vi "save_tiff.vi"(9 "image_info":T1={"file_path"=path "", "file_name"="", "image"=[], "image_size_xy"={"image_size_x_um"=1.0, "image_size_y_um"=1.0}, "pixel_dwell_time_ms"=1.0, "Laser_power_mW"=1.0, "pixel_size"=0.0, "tile_ij"={"tile_i"=0, "tile_j"=0}, "Objective"="", "ColorMarkers"=[], "timestamp"=timestamp(0 s since 1904-01-01), "micro-position-xyz"={"micro-position_x_mm"=1.0, "micro-position_y_mm"=1.0, "micro-position_z_mm"=1.0}, "zero_xyz"={"zero_x_mm"=0.0, "zero_y_mm"=0.0, "zero_z_mm"=0.0}, "nano-position-xyz"={"nano-position_x_V"=1.0, "nano-position_y_V"=1.0, "nano-position_z_V"=1.0}, "Kxyz"={"Kx_V/um"=1.0, "Ky_V/um"=1.0, "Kz_V/um"=1.0}}, 10 "image_array":sgl[][](array[numeric])) -> ()   [LabVIEW 2018]
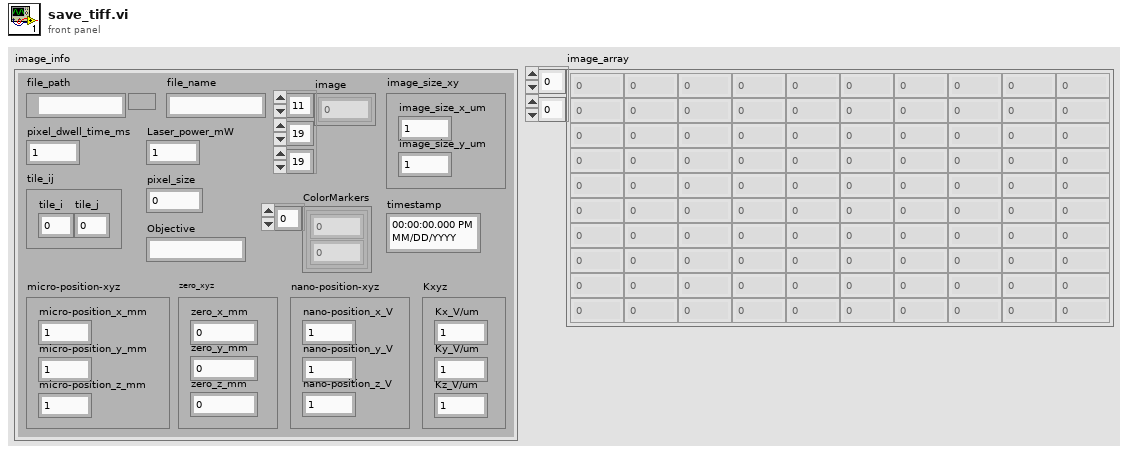
[diagram p1: front panel]
types:
  T1 = cluster{"file_path":path, "file_name":string, "image":dbl[][][], "image_size_xy":cluster{"image_size_x_um":sgl, "image_size_y_um":sgl}, "pixel_dwell_time_ms":sgl, "Laser_power_mW":sgl, "pixel_size":dbl, "tile_ij":cluster{"tile_i":i32, "tile_j":i32}, "Objective":string, "ColorMarkers":cluster{dbl, u32}[], "timestamp":timestamp, "micro-position-xyz":cluster{"micro-position_x_mm":sgl, "micro-position_y_mm":sgl, "micro-position_z_mm":sgl}, "zero_xyz":cluster{"zero_x_mm":dbl, "zero_y_mm":dbl, "zero_z_mm":dbl}, "nano-position-xyz":cluster{"nano-position_x_V":sgl, "nano-position_y_V":sgl, "nano-position_z_V":sgl}, "Kxyz":cluster{"Kx_V/um":sgl, "Ky_V/um":sgl, "Kz_V/um":sgl}}
  T2 = enum16{"open", "replace", "create", "open or create", "replace or create", "replace or create with confirmation"}
  T3 = enum16{"micro-position X", "micro-position Y", "micro-position Z", "nano-position X", "nano-position Y", "nano-position Z", "Pixel dwell time", "Kx", "Ky", "Kz", "Objective", "Laser power", "Timestamp", "ColorMarkers"}[]
  T4 = enum16{"ImageWidth", "ImageLength", "BitsPerSample", "Compression", "PhotometricInterpretation", "StripOffsets", "RowsPerStrip", "StripByteCounts", "XResolution", "YResolution", "ResolutionUnit", "ColorMap"}[]
  T5 = enum16{"big-endian, network order", "native, host order", "little-endian"}
  T6 = enum32{"WhiteIsZero", "BlackIsZero", "RGB", "RGB Palette"}
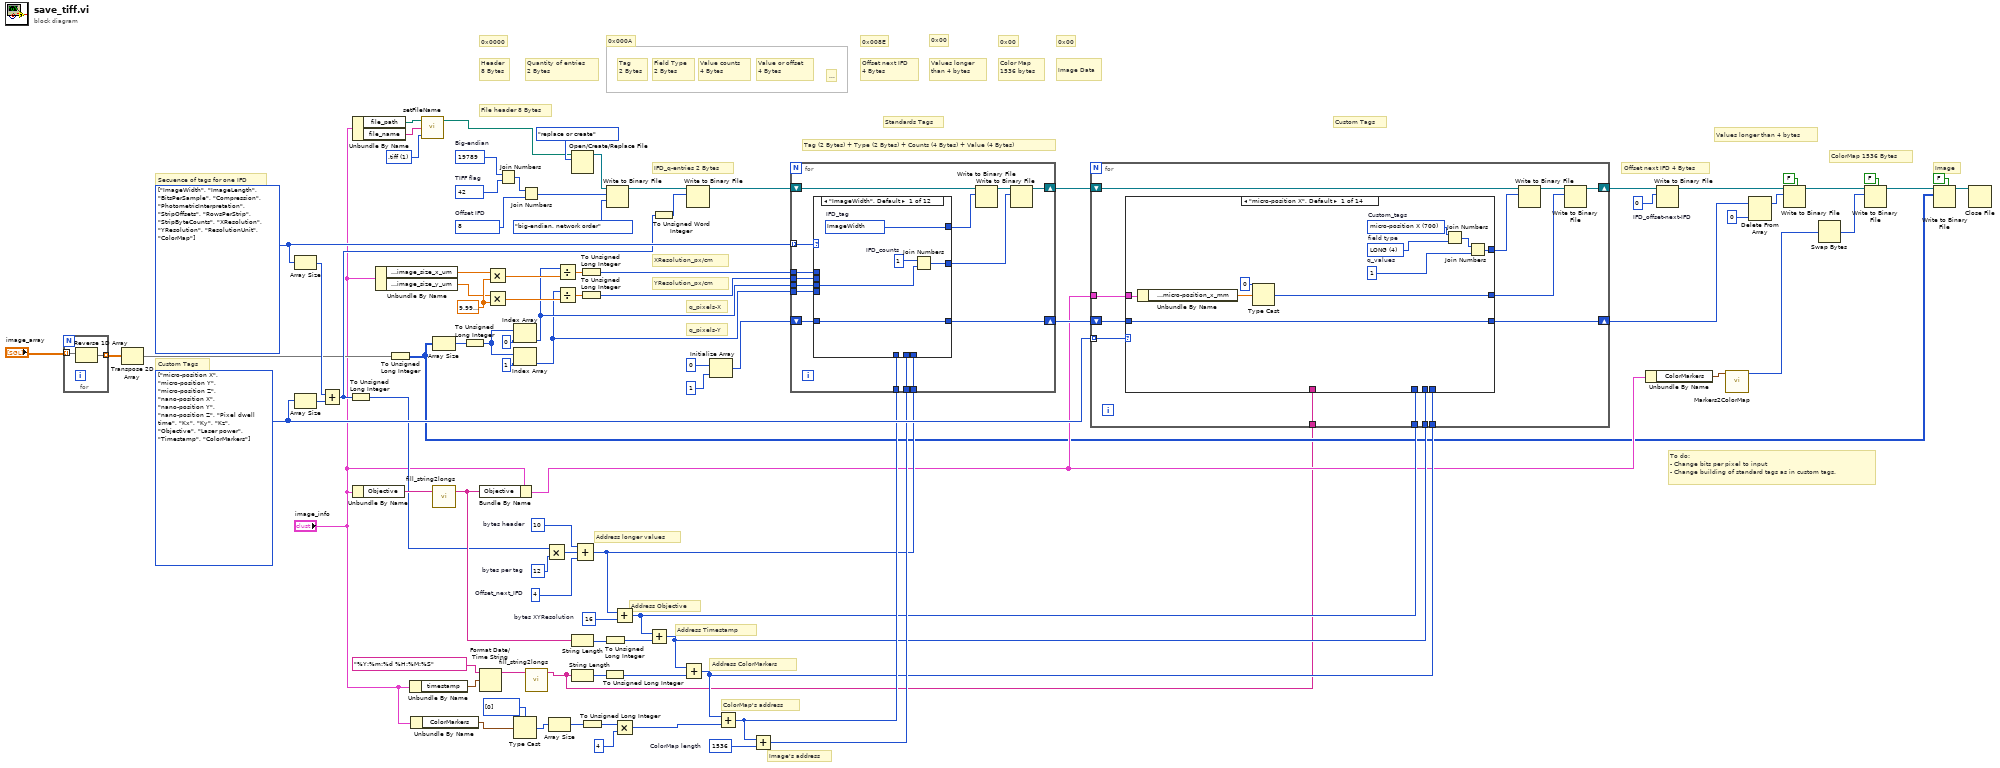
[diagram p0: block diagram]
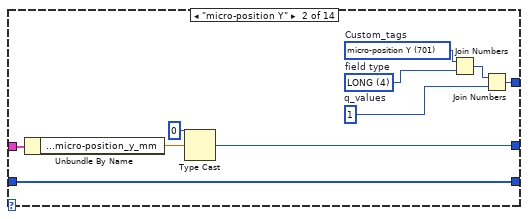
[diagram p2: hidden frame]
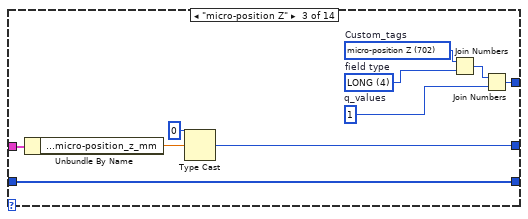
[diagram p3: hidden frame]
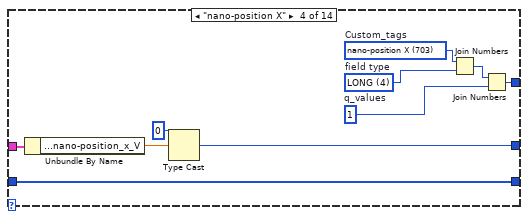
[diagram p4: hidden frame]
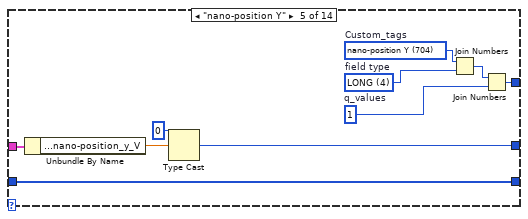
[diagram p5: hidden frame]
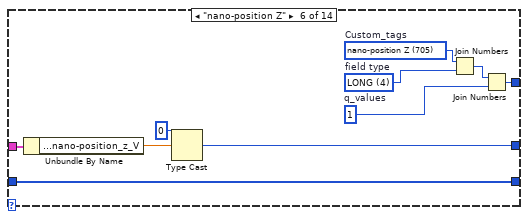
[diagram p6: hidden frame]
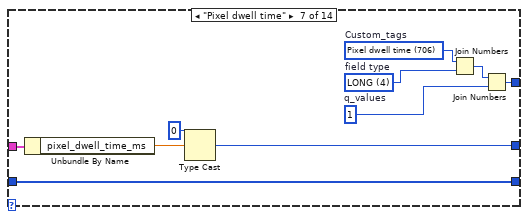
[diagram p7: hidden frame]
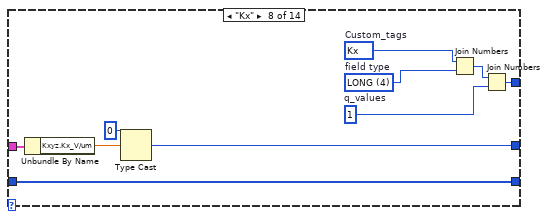
[diagram p8: hidden frame]
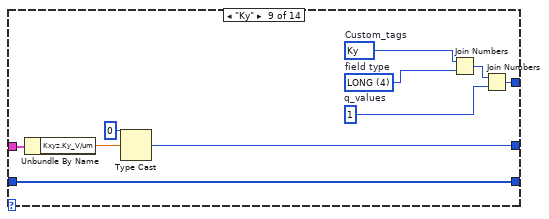
[diagram p9: hidden frame]
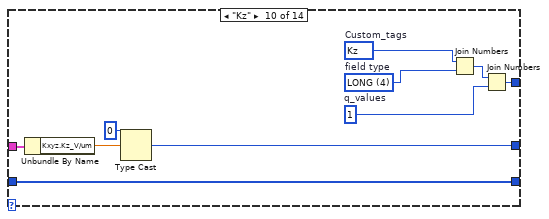
[diagram p10: hidden frame]
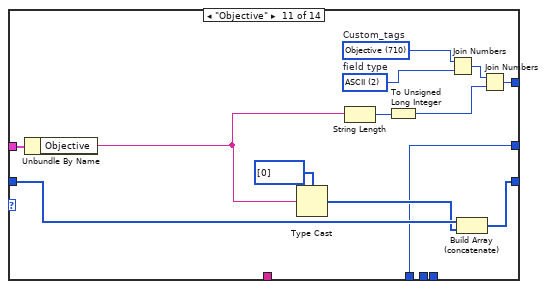
[diagram p11: hidden frame]
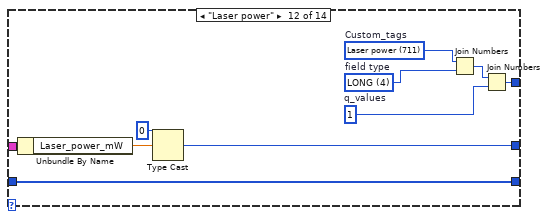
[diagram p12: hidden frame]
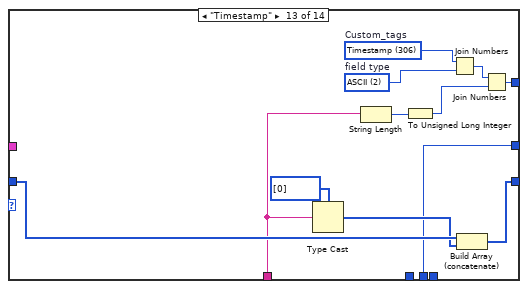
[diagram p13: hidden frame]
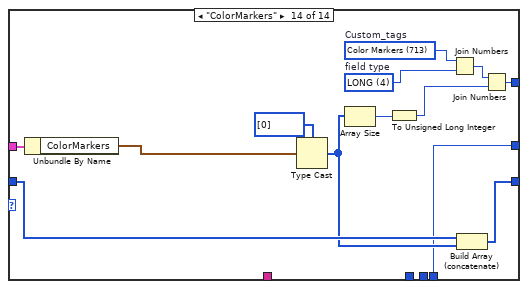
[diagram p14: hidden frame]
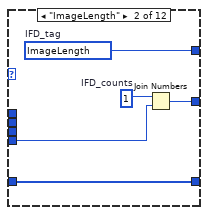
[diagram p15: hidden frame]
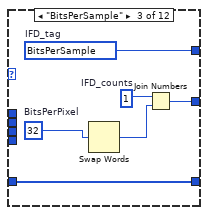
[diagram p16: hidden frame]
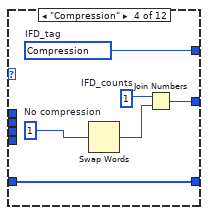
[diagram p17: hidden frame]
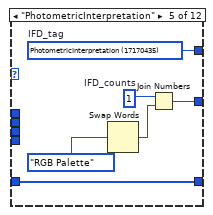
[diagram p18: hidden frame]
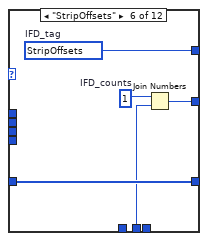
[diagram p19: hidden frame]
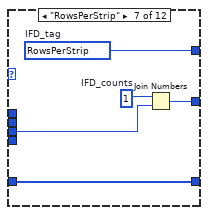
[diagram p20: hidden frame]
diagram:
  w1 = u16 1 items=[".txt", ".tiff"] ("extension")
  w27 = u32 1536  # ColorMap length
  w53 = u32 4  # Offset_next_IFD
  w36 = u32 16  # bytes XYResolution
  w55 = u32 10  # bytes header
  w57 = u32 12  # bytes per tag
  w40 = T3 [enum."micro-position X", enum."micro-position Y", enum."micro-position Z", enum."nano-position X", enum."nano-position Y", enum."nano-position Z", enum."Pixel dwell time", enum."Kx", enum."Ky", enum."Kz", enum."Objective", enum."Laser power", enum."Timestamp", enum."ColorMarkers"] items=["micro-position X", "micro-position Y", "micro-position Z", "nano-position X", "nano-position Y", "nano-position Z", "Pixel dwell time", "Kx", "Ky", "Kz", "Objective", "Laser power", "Timestamp", "ColorMarkers"] ("Custom Tags")
  w73 = sgl 0.0001 ("y")
  w41 = T4 [enum."ImageWidth", enum."ImageLength", enum."BitsPerSample", enum."Compression", enum."PhotometricInterpretation", enum."StripOffsets", enum."RowsPerStrip", enum."StripByteCounts", enum."XResolution", enum."YResolution", enum."ResolutionUnit", enum."ColorMap"] items=["ImageWidth", "ImageLength", "BitsPerSample", "Compression", "PhotometricInterpretation", "StripOffsets", "RowsPerStrip", "StripByteCounts", "XResolution", "YResolution", "ResolutionUnit", "ColorMap"]
  w84 = u32 0  # IFD_offset-next-IFD
  w86 = u16 8  # Offset IFD
  w90 = u16 42  # TIFF flag
  w91 = u16 19789  # Big-endian
  # "Image's address"
  # "Address ColorMarkers"
  # "Address Timestamp"
  # "Address Objective"
  # "To do:\n- Change bits per pixel to input\n- Change building of standard tags as in custom tags."
  # "0x00"
  # "Color Map\n1536 bytes"
  # "ColorMap 1536 Bytes"
  # "Address longer values"
  # "ColorMap's address"
  # "Custom Tags"
  # "Custom Tags"
  # "Standards Tags"
  # "YResolution_px/cm"
  # "XResolution_px/cm"
  # "q_pixels-Y"
  # "q_pixels-X"
  # "Values longer than 4 bytes"
  # "0x00"
  # "Values longer than 4 bytes"
  # "Image"
  # "0x00"
  # "0x008E"
  # "0x000A"
  # "0x0000"
  # "Image Data"
  # "..."
  # "Offset next IFD\n4 Bytes"
  # "Quantity of entries\n2 Bytes"
  # "Value or offset\n4 Bytes"
  # "Value counts\n4 Bytes"
  # "Field Type\n2 Bytes"
  # "Tag\n2 Bytes"
  # "Header\n8 Bytes"
  # "Offset next IFD 4 Bytes"
  # "Tag (2 Bytes) + Type (2 Bytes) + Counts (4 Bytes) + Value (4 Bytes)"
  # "IFD_q-entries 2 Bytes"
  # "Secuence of tags for one IFD"
  # "File header 8 Bytes"
  n1 = for {
    tunnel: "image_array" -> [w93] mode=indexing
    tunnel: [w92] -> w8 mode=indexing
    n2 = Reverse 1D Array(array=w93) -> (reversed array=w92:sgl[])
  }
  n3 = Transpose 2D Array(2D array=w8) -> (transposed array=w7:sgl[][])
  n4 = Array Size(array=w41) -> (size(s)=w38:i32)
  n5 = Array Size(array=w40) -> (size(s)=w39:i32)
  n6 = Add(x=w38, y=w39) -> (x+y=w17:i32)
  n7 = To Unsigned Long Integer(number=w17) -> (unsigned 32bit integer=w37:u32)
  n8 = Unbundle By Name("image_info") -> ("file_path"=w4:path, "file_name"=w3:string)
  n9 = Unbundle By Name("image_info") -> ("Objective"=w54:string)
  n10 = Unbundle By Name("image_info") -> ("image_size_xy.image_size_x_um"=w62:sgl, "image_size_xy.image_size_y_um"=w61:sgl)
  n11 = To Unsigned Long Integer(number=w7) -> (unsigned 32bit integer=w18:u32[][])
  n12 = Unbundle By Name("image_info") -> ("timestamp"=w49:timestamp)
  n13 = Unbundle By Name("image_info") -> ("ColorMarkers"=w31:cluster{dbl, u32}[])
  n14 = call "setFileName.vi"("extension"=w1, "file_name"=w3, "base_path"=w4) -> ("path_filename"=w2:path)  [unwired: 2 in]
  n15 = Array Size(array=w18) -> (size(s)=w77:i32[])
  n16 = call "fill_string2longs.vi"("string_in"=w54) -> ("string_out"=w52:string)  [unwired: 10 in]
  n17 = To Unsigned Long Integer(number=w77) -> (unsigned 32bit integer=w74:u32[])
  n18 = Bundle By Name(cluster="image_info", "Objective"=w52) -> (w20:T1)
  n19 = Format Date/Time String(time format string (%c)="%Y:%m:%d %H:%M:%S", seconds (now)=w49) -> (date/time string=w50:string)  [unwired: 1 in]
  n20 = Multiply(x=w62, y=w73) -> (x*y=w72:sgl)
  n21 = Multiply(x=w61, y=w73) -> (x*y=w71:sgl)
  n22 = Join Numbers(hi=w91, lo=w90) -> ((hi.lo)=w87:u32)
  n23 = Index Array(array=w74, index=0) -> (element=w11:u32)
  n24 = Index Array(array=w74, index=1) -> (element=w10:u32)
  n25 = Type Cast(type=u32[] [0], x=w31) -> (*(type *) &x=w32:u32[])
  n26 = Join Numbers(hi=w87, lo=w86) -> ((hi.lo)=w88:u64)
  n27 = call "fill_string2longs.vi"("string_in"=w50) -> ("string_out"=w6:string)  [unwired: 10 in]
  n28 = Multiply(x=w37, y=w57) -> (x*y=w56:u32)
  n29 = Array Size(array=w32) -> (size(s)=w30:i32)
  n30 = Divide(x=w11, y=w72) -> (x/y=w70:sgl)
  n31 = Divide(x=w10, y=w71) -> (x/y=w69:sgl)
  n32 = Open/Create/Replace File(file path (use dialog)=w2, operation (0:open)=T2."replace or create") -> (refnum out=w59:refnum<file>)  [unwired: 4 in, 2 out]
  n33 = String Length(string=w52) -> (length=w35:i32)
  n34 = String Length(string=w6) -> (length=w34:i32)
  n35 = Compound Arithmetic op=unknown(w55, w56, w53) -> (w24:u32)
  n36 = To Unsigned Long Integer(number=w70) -> (unsigned 32bit integer=w68:u32)
  n37 = To Unsigned Long Integer(number=w69) -> (unsigned 32bit integer=w67:u32)
  n38 = To Unsigned Long Integer(number=w30) -> (unsigned 32bit integer=w14:u32)
  n39 = To Unsigned Long Integer(number=w34) -> (unsigned 32bit integer=w28:u32)
  n40 = To Unsigned Long Integer(number=w35) -> (unsigned 32bit integer=w29:u32)
  n41 = Write to Binary File(file (use dialog)=w59, data=w88, 9:T5."big-endian, network order" ("byte order (0:big-endian, network order)")) -> (refnum out=w85:refnum<file>)  [unwired: 3 in, 2 out]
  n42 = Add(x=w24, y=w36) -> (x+y=w23:u32)
  n43 = Multiply(x=w14, y=u32 4 ("unsigned 32bit integer")) -> (x*y=w15:u32)
  n44 = Add(x=w23, y=w29) -> (x+y=w22:u32)
  n45 = To Unsigned Word Integer(number=w17) -> (unsigned 16bit integer=w16:u16)
  n46 = Add(x=w22, y=w28) -> (x+y=w21:u32)
  n47 = Write to Binary File(file (use dialog)=w85, data=w16) -> (refnum out=w83:refnum<file>)  [unwired: 4 in, 2 out]
  n48 = Initialize Array(u32 0 ("element"), 1 ("dimension size")) -> (w82:u32[])
  n49 = Add(x=w21, y=w15) -> (x+y=w25:u32)
  n50 = Add(x=w25, y=w27) -> (x+y=w26:u32)
  n51 = for {
    tunnel: w41 -> [w108] mode=indexing
    shift-right: [w104] -> w66
    shift-left: w83 -> [w103]
    tunnel: w68 -> [w102]
    tunnel: w67 -> [w101]
    tunnel: w11 -> [w100]
    tunnel: w10 -> [w99]
    shift-right: [w97] -> w63
    shift-left: w82 -> [w98]
    tunnel: w26 -> [w96]
    tunnel: w25 -> [w95]
    tunnel: w24 -> [w94]
    n52 = case shown="\"ImageWidth\", Default" w108 {
      tunnel: [w112 w117 w123 w129 w135 w139 w145 w152 w161 w171 w177 w181] -> w107
      tunnel: [w111 w116 w122 w128 w134 w140 w144 w153 w160 w170 w176 w182] -> w106
      tunnel: w102 -> [_ _ _ _ _ _ _ _ w157 _ _ _]
      tunnel: w101 -> [_ _ _ _ _ _ _ _ _ w167 _ _]
      tunnel: w100 -> [w110 _ _ _ _ _ w143 w149 _ _ _ _]
      tunnel: w99 -> [_ w115 _ _ _ _ _ w150 _ _ _ _]
      tunnel: [w109 w114 w119 w125 w131 w138 w142 w147 w159 w166 w173 w180] -> w97
      tunnel: w98 -> [w109 w114 w119 w125 w131 w138 w142 w147 w158 w169 w173 w180]
      tunnel: w96 -> [_ _ _ _ _ w137 _ _ _ _ _ _]
      tunnel: w95 -> [_ _ _ _ _ _ _ _ _ _ _ w179]
      tunnel: w94 -> [_ _ _ _ _ _ _ _ w155 w164 _ _]
      frame "ImageWidth", Default {
        w112 = u32 16777220 items=["ImageWidth"=16777220, "ImageLength"=16842756, "BitsPerSample"=16908291, "Compression"=16973827, "PhotometricInterpretation"=17170435, "StripOffsets"=17891332, "RowsPerStrip"=18219012, "StripByteCounts"=18284548, "XResolution"=18481157, "YResolution"=18546693, "ResolutionUnit"=19398659]  # IFD_tag
        w113 = u32 1  # IFD_counts
        n53 = Join Numbers(hi=w113, lo=w110) -> ((hi.lo)=w111:u64)
      }
      frame "ImageLength" {
        w117 = u32 16842756 items=["ImageWidth"=16777220, "ImageLength"=16842756, "BitsPerSample"=16908291, "Compression"=16973827, "PhotometricInterpretation"=17170435, "StripOffsets"=17891332, "RowsPerStrip"=18219012, "StripByteCounts"=18284548, "XResolution"=18481157, "YResolution"=18546693, "ResolutionUnit"=19398659]  # IFD_tag
        w118 = u32 1  # IFD_counts
        n54 = Join Numbers(hi=w118, lo=w115) -> ((hi.lo)=w116:u64)
      }
      frame "BitsPerSample" {
        w120 = u32 32  # BitsPerPixel
        w123 = u32 16908291 items=["ImageWidth"=16777220, "ImageLength"=16842756, "BitsPerSample"=16908291, "Compression"=16973827, "PhotometricInterpretation"=17170435, "StripOffsets"=17891332, "RowsPerStrip"=18219012, "StripByteCounts"=18284548, "XResolution"=18481157, "YResolution"=18546693, "ResolutionUnit"=19398659]  # IFD_tag
        w124 = u32 1  # IFD_counts
        n55 = Swap Words(1:w120) -> (0:w121:u32)
        n56 = Join Numbers(hi=w124, lo=w121) -> ((hi.lo)=w122:u64)
      }
      frame "Compression" {
        w127 = u32 1  # No compression
        w129 = u32 16973827 items=["ImageWidth"=16777220, "ImageLength"=16842756, "BitsPerSample"=16908291, "Compression"=16973827, "PhotometricInterpretation"=17170435, "StripOffsets"=17891332, "RowsPerStrip"=18219012, "StripByteCounts"=18284548, "XResolution"=18481157, "YResolution"=18546693, "ResolutionUnit"=19398659]  # IFD_tag
        w130 = u32 1  # IFD_counts
        n57 = Swap Words(1:w127) -> (0:w126:u32)
        n58 = Join Numbers(hi=w130, lo=w126) -> ((hi.lo)=w128:u64)
      }
      frame "PhotometricInterpretation" {
        w135 = u32 17170435 items=["ImageWidth"=16777220, "ImageLength"=16842756, "BitsPerSample"=16908291, "Compression"=16973827, "PhotometricInterpretation"=17170435, "StripOffsets"=17891332, "RowsPerStrip"=18219012, "StripByteCounts"=18284548, "XResolution"=18481157, "YResolution"=18546693, "ResolutionUnit"=19398659]  # IFD_tag
        w136 = u32 1  # IFD_counts
        n59 = Swap Words(1:T6."RGB Palette") -> (0:w132:u32)
        n60 = Join Numbers(hi=w136, lo=w132) -> ((hi.lo)=w134:u64)
      }
      frame "StripOffsets" {
        w139 = u32 17891332 items=["ImageWidth"=16777220, "ImageLength"=16842756, "BitsPerSample"=16908291, "Compression"=16973827, "PhotometricInterpretation"=17170435, "StripOffsets"=17891332, "RowsPerStrip"=18219012, "StripByteCounts"=18284548, "XResolution"=18481157, "YResolution"=18546693, "ResolutionUnit"=19398659]  # IFD_tag
        w141 = u32 1  # IFD_counts
        n61 = Join Numbers(hi=w141, lo=w137) -> ((hi.lo)=w140:u64)
      }
      frame "RowsPerStrip" {
        w145 = u32 18219012 items=["ImageWidth"=16777220, "ImageLength"=16842756, "BitsPerSample"=16908291, "Compression"=16973827, "PhotometricInterpretation"=17170435, "StripOffsets"=17891332, "RowsPerStrip"=18219012, "StripByteCounts"=18284548, "XResolution"=18481157, "YResolution"=18546693, "ResolutionUnit"=19398659]  # IFD_tag
        w146 = u32 1  # IFD_counts
        n62 = Join Numbers(hi=w146, lo=w143) -> ((hi.lo)=w144:u64)
      }
      frame "StripByteCounts" {
        w151 = u32 4  # Bytes per pixel
        w152 = u32 18284548 items=["ImageWidth"=16777220, "ImageLength"=16842756, "BitsPerSample"=16908291, "Compression"=16973827, "PhotometricInterpretation"=17170435, "StripOffsets"=17891332, "RowsPerStrip"=18219012, "StripByteCounts"=18284548, "XResolution"=18481157, "YResolution"=18546693, "ResolutionUnit"=19398659]  # IFD_tag
        w154 = u32 1  # IFD_counts
        n63 = Compound Arithmetic op=MULTIPLY(w151, w149, w150) -> (w148:u32)
        n64 = Join Numbers(hi=w154, lo=w148) -> ((hi.lo)=w153:u64)
      }
      frame "XResolution" {
        w161 = u32 18481157 items=["ImageWidth"=16777220, "ImageLength"=16842756, "BitsPerSample"=16908291, "Compression"=16973827, "PhotometricInterpretation"=17170435, "StripOffsets"=17891332, "RowsPerStrip"=18219012, "StripByteCounts"=18284548, "XResolution"=18481157, "YResolution"=18546693, "ResolutionUnit"=19398659]  # IFD_tag
        w162 = u32 1  # IFD_counts
        n65 = Build Array (concatenate)(w158, w157, u32 1 ("lo")) -> (w159:u32[])
        n66 = Join Numbers(hi=w162, lo=w155) -> ((hi.lo)=w160:u64)
      }
      frame "YResolution" {
        w163 = u32 8  # size_Xres
        w171 = u32 18546693 items=["ImageWidth"=16777220, "ImageLength"=16842756, "BitsPerSample"=16908291, "Compression"=16973827, "PhotometricInterpretation"=17170435, "StripOffsets"=17891332, "RowsPerStrip"=18219012, "StripByteCounts"=18284548, "XResolution"=18481157, "YResolution"=18546693, "ResolutionUnit"=19398659]  # IFD_tag
        w172 = u32 1  # IFD_counts
        n67 = Build Array (concatenate)(w169, w167, u32 1 ("lo")) -> (w166:u32[])
        n68 = Add(x=w163, y=w164) -> (x+y=w165:u32)
        n69 = Join Numbers(hi=w172, lo=w165) -> ((hi.lo)=w170:u64)
      }
      frame "ResolutionUnit" {
        w175 = u32 3 items=["No Unit"=1, "Inch"=2, "Centimeter"=3]
        w177 = u32 19398659 items=["ImageWidth"=16777220, "ImageLength"=16842756, "BitsPerSample"=16908291, "Compression"=16973827, "PhotometricInterpretation"=17170435, "StripOffsets"=17891332, "RowsPerStrip"=18219012, "StripByteCounts"=18284548, "XResolution"=18481157, "YResolution"=18546693, "ResolutionUnit"=19398659]  # IFD_tag
        w178 = u32 1  # IFD_counts
        n70 = Swap Words(1:w175) -> (0:w174:u32)
        n71 = Join Numbers(hi=w178, lo=w174) -> ((hi.lo)=w176:u64)
      }
      frame "ColorMap" {
        w181 = u32 20971523 items=["ImageWidth"=16777220, "ImageLength"=16842756, "BitsPerSample"=16908291, "Compression"=16973827, "PhotometricInterpretation"=17170435, "StripOffsets"=17891332, "RowsPerStrip"=18219012, "StripByteCounts"=18284548, "XResolution"=18481157, "YResolution"=18546693, "ResolutionUnit"=19398659, "ColorMap"=20971523]  # IFD_tag
        w183 = u32 768  # IFD_counts
        n72 = Join Numbers(hi=w183, lo=w179) -> ((hi.lo)=w182:u64)
      }
    }
    n73 = Write to Binary File(file (use dialog)=w103, data=w107) -> (refnum out=w105:refnum<file>)  [unwired: 4 in, 2 out]
    n74 = Write to Binary File(file (use dialog)=w105, data=w106) -> (refnum out=w104:refnum<file>)  [unwired: 4 in, 2 out]
  }
  n75 = for {
    tunnel: w40 -> [w196] mode=indexing
    shift-right: [w192] -> w65
    shift-left: w66 -> [w194]
    shift-right: [w188] -> w64
    shift-left: w63 -> [w195]
    tunnel: w20 -> [w190]
    tunnel: w23 -> [w187]
    tunnel: w22 -> [w186]
    tunnel: w21 -> [w185]
    tunnel: w6 -> [w184]
    n76 = case shown="\"micro-position X\", Default" w196 {
      tunnel: [w202 w216 w220 w230 w240 w250 w260 w270 w280 w290 w302 w313 w326 w343] -> w188
      tunnel: w195 -> [w202 w216 w220 w230 w240 w250 w260 w270 w280 w290 w303 w313 w327 w342]
      tunnel: [w203 w210 w222 w232 w242 w252 w262 w272 w282 w292 w306 w315 w328 w339] -> w193
      tunnel: w190 -> [w200 w211 w221 w231 w241 w251 w261 w271 w281 w291 w305 w314 _ w344]
      tunnel: [w198 w208 w218 w228 w238 w247 w258 w268 w277 w287 w299 w310 w322 w333] -> w189
      tunnel: w187 -> [_ _ _ _ _ _ _ _ _ _ w299 _ _ _]
      tunnel: w186 -> [_ _ _ _ _ _ _ _ _ _ _ _ w322 _]
      tunnel: w185 -> [_ _ _ _ _ _ _ _ _ _ _ _ _ w333]
      tunnel: w184 -> [_ _ _ _ _ _ _ _ _ _ _ _ w320 _]
      frame "micro-position X", Default {
        w201 = u16 700 items=["micro-position X"=700, "micro-position Y"=701, "micro-position Z"=702, "nano-position X"=703, "nano-position Y"=704, "nano-position Z"=705, "Pixel dwell time"=706, "Kx"=707, "Ky"=708, "Kz"=709, "Objective"=710, "Laser power"=711, "Timestamp"=712]  # Custom_tags
        w204 = u32 1  # q_values
        w206 = u16 4 items=["Byte"=1, "ASCII"=2, "SHORT"=3, "LONG"=4, "RATIONAL"=5]  # field type
        n77 = Unbundle By Name(w200) -> ("micro-position-xyz.micro-position_x_mm"=w197:sgl)
        n78 = Type Cast(type=u32 0, x=w197) -> (*(type *) &x=w198:u32)
        n79 = Join Numbers(hi=w201, lo=w206) -> ((hi.lo)=w205:u32)
        n80 = Join Numbers(hi=w205, lo=w204) -> ((hi.lo)=w203:u64)
      }
      frame "micro-position Y" {
        w215 = u16 701 items=["micro-position X"=700, "micro-position Y"=701, "micro-position Z"=702, "nano-position X"=703, "nano-position Y"=704, "nano-position Z"=705, "Pixel dwell time"=706, "Kx"=707, "Ky"=708, "Kz"=709, "Objective"=710, "Laser power"=711, "Timestamp"=712]  # Custom_tags
        w214 = u32 1  # q_values
        w212 = u16 4 items=["Byte"=1, "ASCII"=2, "SHORT"=3, "LONG"=4, "RATIONAL"=5]  # field type
        n81 = Unbundle By Name(w211) -> ("micro-position-xyz.micro-position_y_mm"=w207:sgl)
        n82 = Type Cast(type=u32 0, x=w207) -> (*(type *) &x=w208:u32)
        n83 = Join Numbers(hi=w215, lo=w212) -> ((hi.lo)=w213:u32)
        n84 = Join Numbers(hi=w213, lo=w214) -> ((hi.lo)=w210:u64)
      }
      frame "micro-position Z" {
        w226 = u16 702 items=["micro-position X"=700, "micro-position Y"=701, "micro-position Z"=702, "nano-position X"=703, "nano-position Y"=704, "nano-position Z"=705, "Pixel dwell time"=706, "Kx"=707, "Ky"=708, "Kz"=709, "Objective"=710, "Laser power"=711, "Timestamp"=712]  # Custom_tags
        w225 = u32 1  # q_values
        w223 = u16 4 items=["Byte"=1, "ASCII"=2, "SHORT"=3, "LONG"=4, "RATIONAL"=5]  # field type
        n85 = Unbundle By Name(w221) -> ("micro-position-xyz.micro-position_z_mm"=w217:sgl)
        n86 = Type Cast(type=u32 0, x=w217) -> (*(type *) &x=w218:u32)
        n87 = Join Numbers(hi=w226, lo=w223) -> ((hi.lo)=w224:u32)
        n88 = Join Numbers(hi=w224, lo=w225) -> ((hi.lo)=w222:u64)
      }
      frame "nano-position X" {
        w236 = u16 703 items=["micro-position X"=700, "micro-position Y"=701, "micro-position Z"=702, "nano-position X"=703, "nano-position Y"=704, "nano-position Z"=705, "Pixel dwell time"=706, "Kx"=707, "Ky"=708, "Kz"=709, "Objective"=710, "Laser power"=711, "Timestamp"=712]  # Custom_tags
        w235 = u32 1  # q_values
        w233 = u16 4 items=["Byte"=1, "ASCII"=2, "SHORT"=3, "LONG"=4, "RATIONAL"=5]  # field type
        n89 = Unbundle By Name(w231) -> ("nano-position-xyz.nano-position_x_V"=w227:sgl)
        n90 = Type Cast(type=u32 0, x=w227) -> (*(type *) &x=w228:u32)
        n91 = Join Numbers(hi=w236, lo=w233) -> ((hi.lo)=w234:u32)
        n92 = Join Numbers(hi=w234, lo=w235) -> ((hi.lo)=w232:u64)
      }
      frame "nano-position Y" {
        w246 = u16 704 items=["micro-position X"=700, "micro-position Y"=701, "micro-position Z"=702, "nano-position X"=703, "nano-position Y"=704, "nano-position Z"=705, "Pixel dwell time"=706, "Kx"=707, "Ky"=708, "Kz"=709, "Objective"=710, "Laser power"=711, "Timestamp"=712]  # Custom_tags
        w245 = u32 1  # q_values
        w243 = u16 4 items=["Byte"=1, "ASCII"=2, "SHORT"=3, "LONG"=4, "RATIONAL"=5]  # field type
        n93 = Unbundle By Name(w241) -> ("nano-position-xyz.nano-position_y_V"=w237:sgl)
        n94 = Type Cast(type=u32 0, x=w237) -> (*(type *) &x=w238:u32)
        n95 = Join Numbers(hi=w246, lo=w243) -> ((hi.lo)=w244:u32)
        n96 = Join Numbers(hi=w244, lo=w245) -> ((hi.lo)=w242:u64)
      }
      frame "nano-position Z" {
        w256 = u16 705 items=["micro-position X"=700, "micro-position Y"=701, "micro-position Z"=702, "nano-position X"=703, "nano-position Y"=704, "nano-position Z"=705, "Pixel dwell time"=706, "Kx"=707, "Ky"=708, "Kz"=709, "Objective"=710, "Laser power"=711, "Timestamp"=712]  # Custom_tags
        w255 = u32 1  # q_values
        w253 = u16 4 items=["Byte"=1, "ASCII"=2, "SHORT"=3, "LONG"=4, "RATIONAL"=5]  # field type
        n97 = Unbundle By Name(w251) -> ("nano-position-xyz.nano-position_z_V"=w248:sgl)
        n98 = Type Cast(type=u32 0, x=w248) -> (*(type *) &x=w247:u32)
        n99 = Join Numbers(hi=w256, lo=w253) -> ((hi.lo)=w254:u32)
        n100 = Join Numbers(hi=w254, lo=w255) -> ((hi.lo)=w252:u64)
      }
      frame "Pixel dwell time" {
        w266 = u16 706 items=["micro-position X"=700, "micro-position Y"=701, "micro-position Z"=702, "nano-position X"=703, "nano-position Y"=704, "nano-position Z"=705, "Pixel dwell time"=706, "Kx"=707, "Ky"=708, "Kz"=709, "Objective"=710, "Laser power"=711, "Timestamp"=712]  # Custom_tags
        w265 = u32 1  # q_values
        w263 = u16 4 items=["Byte"=1, "ASCII"=2, "SHORT"=3, "LONG"=4, "RATIONAL"=5]  # field type
        n101 = Unbundle By Name(w261) -> ("pixel_dwell_time_ms"=w257:sgl)
        n102 = Type Cast(type=u32 0, x=w257) -> (*(type *) &x=w258:u32)
        n103 = Join Numbers(hi=w266, lo=w263) -> ((hi.lo)=w264:u32)
        n104 = Join Numbers(hi=w264, lo=w265) -> ((hi.lo)=w262:u64)
      }
      frame "Kx" {
        w276 = u16 707 items=["micro-position X"=700, "micro-position Y"=701, "micro-position Z"=702, "nano-position X"=703, "nano-position Y"=704, "nano-position Z"=705, "Pixel dwell time"=706, "Kx"=707, "Ky"=708, "Kz"=709, "Objective"=710, "Laser power"=711, "Timestamp"=712]  # Custom_tags
        w275 = u32 1  # q_values
        w273 = u16 4 items=["Byte"=1, "ASCII"=2, "SHORT"=3, "LONG"=4, "RATIONAL"=5]  # field type
        n105 = Unbundle By Name(w271) -> ("Kxyz.Kx_V/um"=w269:sgl)
        n106 = Type Cast(type=u32 0, x=w269) -> (*(type *) &x=w268:u32)
        n107 = Join Numbers(hi=w276, lo=w273) -> ((hi.lo)=w274:u32)
        n108 = Join Numbers(hi=w274, lo=w275) -> ((hi.lo)=w272:u64)
      }
      frame "Ky" {
        w286 = u16 708 items=["micro-position X"=700, "micro-position Y"=701, "micro-position Z"=702, "nano-position X"=703, "nano-position Y"=704, "nano-position Z"=705, "Pixel dwell time"=706, "Kx"=707, "Ky"=708, "Kz"=709, "Objective"=710, "Laser power"=711, "Timestamp"=712]  # Custom_tags
        w285 = u32 1  # q_values
        w283 = u16 4 items=["Byte"=1, "ASCII"=2, "SHORT"=3, "LONG"=4, "RATIONAL"=5]  # field type
        n109 = Unbundle By Name(w281) -> ("Kxyz.Ky_V/um"=w278:sgl)
        n110 = Type Cast(type=u32 0, x=w278) -> (*(type *) &x=w277:u32)
        n111 = Join Numbers(hi=w286, lo=w283) -> ((hi.lo)=w284:u32)
        n112 = Join Numbers(hi=w284, lo=w285) -> ((hi.lo)=w282:u64)
      }
      frame "Kz" {
        w296 = u16 709 items=["micro-position X"=700, "micro-position Y"=701, "micro-position Z"=702, "nano-position X"=703, "nano-position Y"=704, "nano-position Z"=705, "Pixel dwell time"=706, "Kx"=707, "Ky"=708, "Kz"=709, "Objective"=710, "Laser power"=711, "Timestamp"=712]  # Custom_tags
        w295 = u32 1  # q_values
        w293 = u16 4 items=["Byte"=1, "ASCII"=2, "SHORT"=3, "LONG"=4, "RATIONAL"=5]  # field type
        n113 = Unbundle By Name(w291) -> ("Kxyz.Kz_V/um"=w288:sgl)
        n114 = Type Cast(type=u32 0, x=w288) -> (*(type *) &x=w287:u32)
        n115 = Join Numbers(hi=w296, lo=w293) -> ((hi.lo)=w294:u32)
        n116 = Join Numbers(hi=w294, lo=w295) -> ((hi.lo)=w292:u64)
      }
      frame "Objective" {
        w309 = u16 710 items=["micro-position X"=700, "micro-position Y"=701, "micro-position Z"=702, "nano-position X"=703, "nano-position Y"=704, "nano-position Z"=705, "Pixel dwell time"=706, "Kx"=707, "Ky"=708, "Kz"=709, "Objective"=710, "Laser power"=711, "Timestamp"=712]  # Custom_tags
        w307 = u16 2 items=["Byte"=1, "ASCII"=2, "SHORT"=3, "LONG"=4, "RATIONAL"=5]  # field type
        n117 = Unbundle By Name(w305) -> ("Objective"=w297:string)
        n118 = Type Cast(type=u32[] [0], x=w297) -> (*(type *) &x=w300:u32[])
        n119 = String Length(string=w297) -> (length=w298:i32)
        n120 = To Unsigned Long Integer(number=w298) -> (unsigned 32bit integer=w301:u32)
        n121 = Join Numbers(hi=w309, lo=w307) -> ((hi.lo)=w308:u32)
        n122 = Build Array (concatenate)(w303, w300) -> (w302:u32[])
        n123 = Join Numbers(hi=w308, lo=w301) -> ((hi.lo)=w306:u64)
      }
      frame "Laser power" {
        w319 = u16 711 items=["micro-position X"=700, "micro-position Y"=701, "micro-position Z"=702, "nano-position X"=703, "nano-position Y"=704, "nano-position Z"=705, "Pixel dwell time"=706, "Kx"=707, "Ky"=708, "Kz"=709, "Objective"=710, "Laser power"=711, "Timestamp"=712]  # Custom_tags
        w318 = u32 1  # q_values
        w316 = u16 4 items=["Byte"=1, "ASCII"=2, "SHORT"=3, "LONG"=4, "RATIONAL"=5]  # field type
        n124 = Unbundle By Name(w314) -> ("Laser_power_mW"=w311:sgl)
        n125 = Type Cast(type=u32 0, x=w311) -> (*(type *) &x=w310:u32)
        n126 = Join Numbers(hi=w319, lo=w316) -> ((hi.lo)=w317:u32)
        n127 = Join Numbers(hi=w317, lo=w318) -> ((hi.lo)=w315:u64)
      }
      frame "Timestamp" {
        w331 = u16 306 items=["micro-position X"=700, "micro-position Y"=701, "micro-position Z"=702, "nano-position X"=703, "nano-position Y"=704, "nano-position Z"=705, "Pixel dwell time"=706, "Kx"=707, "Ky"=708, "Kz"=709, "Objective"=710, "Laser power"=711, "Timestamp"=306]  # Custom_tags
        w329 = u16 2 items=["Byte"=1, "ASCII"=2, "SHORT"=3, "LONG"=4, "RATIONAL"=5]  # field type
        n128 = Type Cast(type=u32[] [0], x=w320) -> (*(type *) &x=w323:u32[])
        n129 = String Length(string=w320) -> (length=w321:i32)
        n130 = To Unsigned Long Integer(number=w321) -> (unsigned 32bit integer=w324:u32)
        n131 = Join Numbers(hi=w331, lo=w329) -> ((hi.lo)=w330:u32)
        n132 = Build Array (concatenate)(w327, w323) -> (w326:u32[])
        n133 = Join Numbers(hi=w330, lo=w324) -> ((hi.lo)=w328:u64)
      }
      frame "ColorMarkers" {
        w337 = u16 713 items=["micro-position X"=700, "micro-position Y"=701, "micro-position Z"=702, "nano-position X"=703, "nano-position Y"=704, "nano-position Z"=705, "Pixel dwell time"=706, "Kx"=707, "Ky"=708, "Kz"=709, "Objective"=710, "Laser power"=711, "Timestamp"=712, "Color Markers"=713]  # Custom_tags
        w340 = u16 4 items=["Byte"=1, "ASCII"=2, "SHORT"=3, "LONG"=4, "RATIONAL"=5]  # field type
        n134 = Unbundle By Name(w344) -> ("ColorMarkers"=w332:cluster{dbl, u32}[])
        n135 = Type Cast(type=u32[] [0], x=w332) -> (*(type *) &x=w336:u32[])
        n136 = Array Size(array=w336) -> (size(s)=w335:i32)
        n137 = To Unsigned Long Integer(number=w335) -> (unsigned 32bit integer=w334:u32)
        n138 = Join Numbers(hi=w337, lo=w340) -> ((hi.lo)=w341:u32)
        n139 = Build Array (concatenate)(w342, w336) -> (w343:u32[])
        n140 = Join Numbers(hi=w341, lo=w334) -> ((hi.lo)=w339:u64)
      }
    }
    n141 = Write to Binary File(file (use dialog)=w194, data=w193) -> (refnum out=w191:refnum<file>)  [unwired: 4 in, 2 out]
    n142 = Write to Binary File(file (use dialog)=w191, data=w189) -> (refnum out=w192:refnum<file>)  [unwired: 4 in, 2 out]
  }
  n143 = Unbundle By Name(w20) -> ("ColorMarkers"=w19:cluster{dbl, u32}[])
  n144 = Write to Binary File(file (use dialog)=w65, data=w84) -> (refnum out=w78:refnum<file>)  [unwired: 4 in, 2 out]
  n145 = call "Markers2ColorMap.vi"("Markers-colors"=w19) -> ("ColorMap"=w12:u16[])  [unwired: 10 in]
  n146 = Delete From Array(array=w64, index=0) -> (array with subset deleted=w43:u32[])  [unwired: 1 in, 1 out]
  n147 = Write to Binary File(file (use dialog)=w78, data=w43, 5:FALSE ("prepend array or string size? (T)")) -> (refnum out=w46:refnum<file>)  [unwired: 3 in, 2 out]
  n148 = Swap Bytes(anything=w12) -> (byte swapped=w45:u16[])
  n149 = Write to Binary File(file (use dialog)=w46, data=w45, 5:FALSE ("prepend array or string size? (T)")) -> (refnum out=w47:refnum<file>)  [unwired: 3 in, 2 out]
  n150 = Write to Binary File(file (use dialog)=w47, data=w18, 5:FALSE ("prepend array or string size? (T)")) -> (refnum out=w60:refnum<file>)  [unwired: 3 in, 2 out]
  n151 = Close File(refnum=w60) -> ()  [unwired: 1 in, 2 out]
